vi "FlatToRichnixnet_grpc_WriteStateValue.vi"(5 "OutputClusterType":T1, 11 "InputCluster":T2) -> (3 "OutputCluster":T1)   [LabVIEW 2025, in "grpc-xnet_client.lvlib"]
uses:
  nixnet_grpc_WriteStateValue_Flat.ctl
  nixnet_grpc_LinDiagnosticScheduleChangeRequest_Flat.ctl
  nixnet_grpc_LinDiagnosticSchedule.ctl
  nixnet_grpc_WriteStateValue.ctl
  nixnet_grpc_WriteStateValue_value/nixnet_grpc_WriteStateValue_value.lvclass
  grpc-xnet_client.lvlib
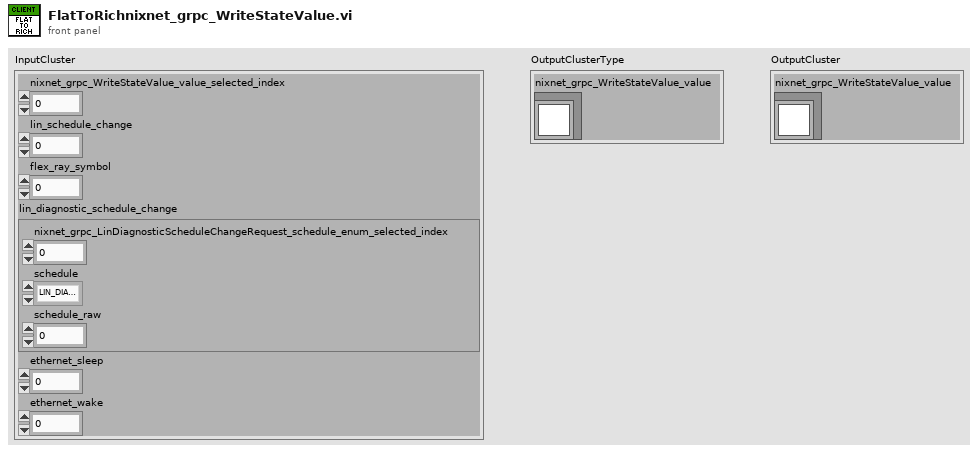
[diagram p1: front panel]
types:
  T1 = typedef "grpc-xnet_client.lvlib/nixnet_grpc_WriteStateValue.ctl" = cluster{"nixnet_grpc_WriteStateValue_value":refnum<class "nixnet_grpc_WriteStateValue_value.lvclass">}
  T2 = typedef "grpc-xnet_client.lvlib/nixnet_grpc_WriteStateValue_Flat.ctl" = cluster{"nixnet_grpc_WriteStateValue_value_selected_index":i32, "lin_schedule_change":u32, "flex_ray_symbol":u32, "lin_diagnostic_schedule_change":T3, "ethernet_sleep":u32, "ethernet_wake":u32}
  T3 = typedef "grpc-xnet_client.lvlib/nixnet_grpc_LinDiagnosticScheduleChangeRequest_Flat.ctl" = cluster{"nixnet_grpc_LinDiagnosticScheduleChangeRequest_schedule_enum_selected_index":i32, "schedule":T4, "schedule_raw":u32}
  T4 = typedef "grpc-xnet_client.lvlib/nixnet_grpc_LinDiagnosticSchedule.ctl" = enum32{"LIN_DIAGNOSTIC_SCHEDULE_NULL", "LIN_DIAGNOSTIC_SCHEDULE_MASTER_REQ", "LIN_DIAGNOSTIC_SCHEDULE_SLAVE_RESP"}
  T5 = typedef "grpc-xnet_client.lvlib/nixnet_grpc_LinDiagnosticScheduleChangeRequest.ctl" = cluster{"nixnet_grpc_LinDiagnosticScheduleChangeRequest_schedule_enum":refnum<class "nixnet_grpc_LinDiagnosticScheduleChangeRequest_schedule_enum.lvclass">}
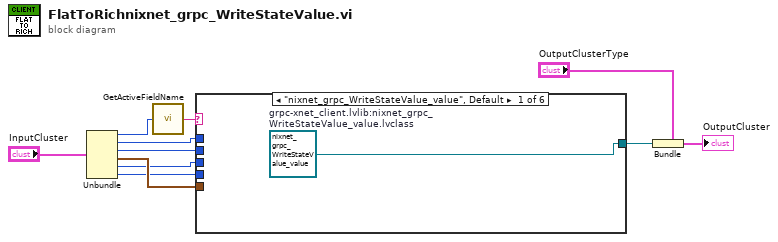
[diagram p0: block diagram]
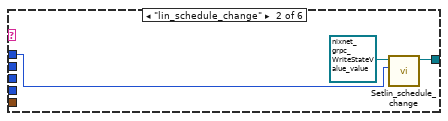
[diagram p2: hidden frame]
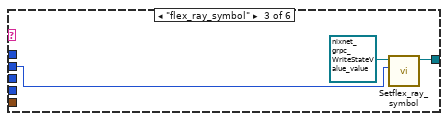
[diagram p3: hidden frame]
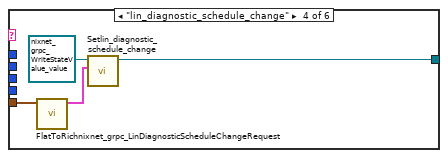
[diagram p4: hidden frame]
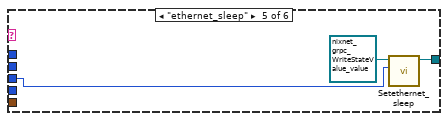
[diagram p5: hidden frame]
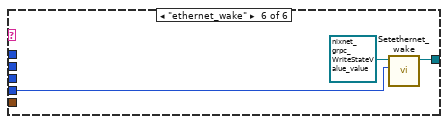
[diagram p6: hidden frame]
diagram:
  n1 = Unbundle "Unbundle"("InputCluster") -> ("nixnet_grpc_WriteStateValue_value_selected_index"=w8:i32, "lin_schedule_change"=w5:u32, "flex_ray_symbol"=w4:u32, "lin_diagnostic_schedule_change"=w3:T3, "ethernet_sleep"=w2:u32, "ethernet_wake"=w1:u32)
  n2 = call "GetActiveFieldName.vi"("protobuf index"=w8) -> ("oneof field name"=w7:string)
  n3 = case "nixnet_grpc_WriteStateValue_value" shown="\"nixnet_grpc_WriteStateValue_value\", Default" w7 {
    tunnel: [w12 w14 w17 w20 w24 w27] -> w6
    tunnel: w5 -> [_ w15 _ _ _ _]
    tunnel: w4 -> [_ _ w18 _ _ _]
    tunnel: w3 -> [_ _ _ w22 _ _]
    tunnel: w2 -> [_ _ _ _ w25 _]
    tunnel: w1 -> [_ _ _ _ _ w28]
    frame "nixnet_grpc_WriteStateValue_value", Default {
      w12 = refnum<class "nixnet_grpc_WriteStateValue_value.lvclass"> refnum  # grpc-xnet_client.lvlib:nixnet_grpc_WriteStateValue_value.lvclass
    }
    frame "lin_schedule_change" {
      n4 = call "Setlin_schedule_change.vi"("Set_Val"=w15, "OneOfTemplate in"=refnum<class "nixnet_grpc_WriteStateValue_value.lvclass"> refnum) -> ("OneOfTemplate out"=w14:refnum<class "nixnet_grpc_WriteStateValue_value.lvclass">)  [unwired: 8 in, 1 out]
    }
    frame "flex_ray_symbol" {
      n5 = call "Setflex_ray_symbol.vi"("Set_Val"=w18, "OneOfTemplate in"=refnum<class "nixnet_grpc_WriteStateValue_value.lvclass"> refnum) -> ("OneOfTemplate out"=w17:refnum<class "nixnet_grpc_WriteStateValue_value.lvclass">)  [unwired: 8 in, 1 out]
    }
    frame "lin_diagnostic_schedule_change" {
      n6 = call "FlatToRichnixnet_grpc_LinDiagnosticScheduleChangeRequest.vi"("InputCluster"=w22) -> ("OutputCluster"=w21:T5)  [unwired: 10 in]
      n7 = call "Setlin_diagnostic_schedule_change.vi"("Set_Val"=w21, "OneOfTemplate in"=refnum<class "nixnet_grpc_WriteStateValue_value.lvclass"> refnum) -> ("OneOfTemplate out"=w20:refnum<class "nixnet_grpc_WriteStateValue_value.lvclass">)  [unwired: 8 in, 1 out]
    }
    frame "ethernet_sleep" {
      n8 = call "Setethernet_sleep.vi"("Set_Val"=w25, "OneOfTemplate in"=refnum<class "nixnet_grpc_WriteStateValue_value.lvclass"> refnum) -> ("OneOfTemplate out"=w24:refnum<class "nixnet_grpc_WriteStateValue_value.lvclass">)  [unwired: 8 in, 1 out]
    }
    frame "ethernet_wake" {
      n9 = call "Setethernet_wake.vi"("Set_Val"=w28, "OneOfTemplate in"=refnum<class "nixnet_grpc_WriteStateValue_value.lvclass"> refnum) -> ("OneOfTemplate out"=w27:refnum<class "nixnet_grpc_WriteStateValue_value.lvclass">)  [unwired: 8 in, 1 out]
    }
  }
  n10 = Bundle "Bundle"(cluster="OutputClusterType", "nixnet_grpc_WriteStateValue_value"=w6) -> (→"OutputCluster":T1)
